vi "Initialize NI-Digital Session.vi"(8 "error in (no error)":errorcluster, 10 "session information":T3, 11 "gRPC clients":T1) -> (0 "error out":errorcluster, 2 "instrument handle":refnum<k15>, 3 "gRPC clients out":T1)   [LabVIEW 2020, in "NIDigitalSPI.lvlib"]
doc: "Creates and returns a gRPC based NI-DCPower instrument handle."
uses:
  NIDigitalSPI.lvlib
  <vilib>/MeasurementLink/MeasurementLink Session Management Client/RPC Messages/ni_measurementlink_sessionmanagement_v1_SessionInformation.ctl
  <vilib>/MeasurementLink/MeasurementLink Session Management Client/RPC Messages/nidevice_grpc_Session.ctl
  <vilib>/MeasurementLink/MeasurementLink Session Management Client/RPC Messages/ni_measurementlink_sessionmanagement_v1_ChannelMapping.ctl
  Measurement Service Helpers/GRPC Clients.ctl
  <vilib>/gRPC/LabVIEW gRPC Library/Shared/grpcId.ctl
  Measurement Service Helpers/Measurement Service Helpers.lvlib
  <vilib>/MeasurementLink/MeasurementLink Session Management Client/MeasurementLink Session Management Client.lvlib
  <vilib>/gRPC/LabVIEW gRPC Library/grpc-lvsupport-release.lvlib
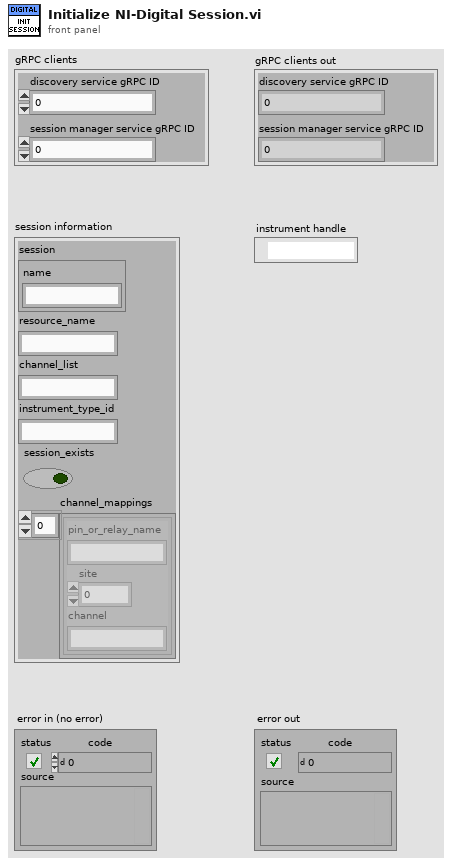
[diagram p1: front panel]
types:
  T1 = typedef "Measurement Service Helpers.lvlib/GRPC Clients.ctl" = cluster{"discovery service gRPC ID":T2, "session manager service gRPC ID":T2}
  T2 = typedef "grpc-lvsupport-release.lvlib/grpcId.ctl" = u64
  T3 = typedef "MeasurementLink Session Management Client.lvlib/ni_measurementlink_sessionmanagement_v1_SessionInformation.ctl" = cluster{"session":T4, "resource_name":string, "channel_list":string, "instrument_type_id":string, "session_exists":bool, "channel_mappings":T5[]}
  T4 = typedef "MeasurementLink Session Management Client.lvlib/nidevice_grpc_Session.ctl" = cluster{"name":string}
  T5 = typedef "MeasurementLink Session Management Client.lvlib/ni_measurementlink_sessionmanagement_v1_ChannelMapping.ctl" = cluster{"pin_or_relay_name":string, "site":i32, "channel":string}
  T6 = typedef "MeasurementLink Discovery Client.lvlib/ni_measurementlink_discovery_v1_ServiceLocation.ctl" = cluster{"location":string, "insecure_port":string, "ssl_authenticated_port":string}
  T7 = typedef "Measurement Service Helpers.lvlib/gRPC Device Options.ctl" = cluster{"session name":string, "address (localhost)":string, "port (31763)":u32}
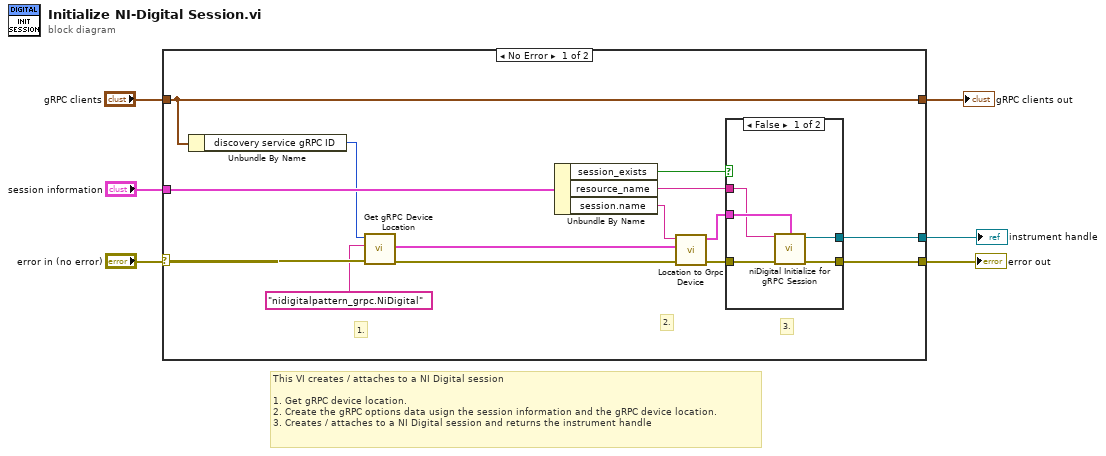
[diagram p0: block diagram]
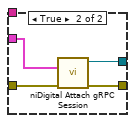
[diagram p2: hidden frame]
diagram:
  # "This VI creates / attaches to a NI Digital session\n\n1. Get gRPC device location.\n2. Create the gRPC options data usign the session information and the gRPC device location.\n3. Creates / attaches to a NI Digital session and returns the instrument handle"
  n1 = case shown="No Error" "error in (no error)" {
    selector: "error in (no error)" -> [w12 w30]
    tunnel: "session information" -> [w19 _]
    tunnel: [w14 w30] -> w5
    tunnel: [w13 _] -> w1
    tunnel: "gRPC clients" -> [w8 w29]
    tunnel: [w8 w29] -> w2
    frame No Error {
      # "3."
      # "2."
      # "1."
      n2 = Unbundle By Name(w8) -> ("discovery service gRPC ID"=w7:T2)
      n3 = call "Get gRPC Device Location.vi"("error in"=w12, "provided_interface"="nidigitalpattern_grpc.NiDigital", "discovery service gRPC ID"=w7) -> ("error out"=w11:errorcluster, "gRPC device location"=w9:T6)  [unwired: 6 in, 1 out]
      n4 = Unbundle By Name(w19) -> ("session_exists"=w18:bool, "resource_name"=w15:string, "session.name"=w17:string)
      n5 = call "Location to Grpc Device.vi"("Grpc Device Location"=w9, "Session Name"=w17) -> ("gRPC Device Options"=w16:T7)  [unwired: 9 in]
      n6 = case shown="False" w18 {
        tunnel: w16 -> [w22 w26]
        tunnel: w15 -> [w21 _]
        tunnel: w11 -> [w24 w28]
        tunnel: [w23 w27] -> w14
        tunnel: [w20 w25] -> w13
        frame False {
          n7 = call <instrlib>:"niDigital Initialize for gRPC Session.vi"("resource name"=w21, "gRPC options"=w22, "error in"=w24) -> ("instrument handle"=w20:refnum<k15>, "error out"=w23:errorcluster)  [unwired: 11 in]
        }
        frame True {
          n8 = call <instrlib>:"niDigital Attach gRPC Session.vi"("gRPC options"=w26, "error in"=w28) -> ("instrument handle out"=w25:refnum<k15>, "error out"=w27:errorcluster)  [unwired: 12 in]
        }
      }
    }
    frame Error {
    }
  }
  "error out" <- w5
  "gRPC clients out" <- w2
  "instrument handle" <- w1
